vi "util.filter-rec-files-by-date.vi"(9 "Date Start":timestamp format="%<%x>T", 10 "Date End":timestamp format="%<%x>T", 11 "filenames":string[](array[string])) -> (0 "error IO":errorcluster, 3 "Array":string[](array[string]))   [LabVIEW 2024]
uses:
  <vilib>/Utility/miscctls.llb/LVDateTimeRec.ctl
panel:
  out "double precision float":dbl format="%#.0f"
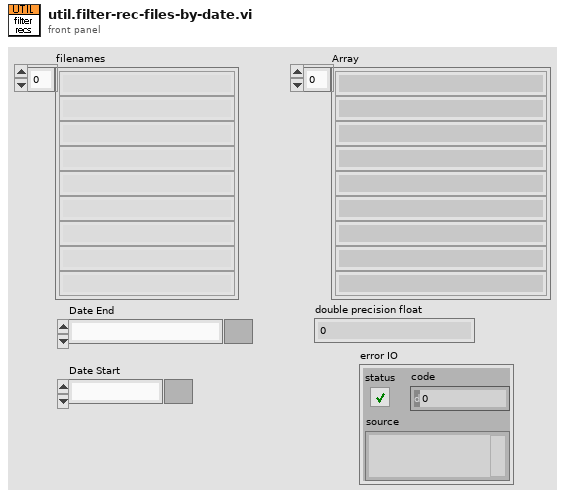
[diagram p1: front panel]
types:
  T1 = typedef "LVDateTimeRec.ctl" = cluster{"fractional second":dbl, "second":i32, "minute":i32, "hour":i32, "day of month":i32, "month":i32, "year":i32, "day of week":i32, "day of year":i32, "DST":i32}
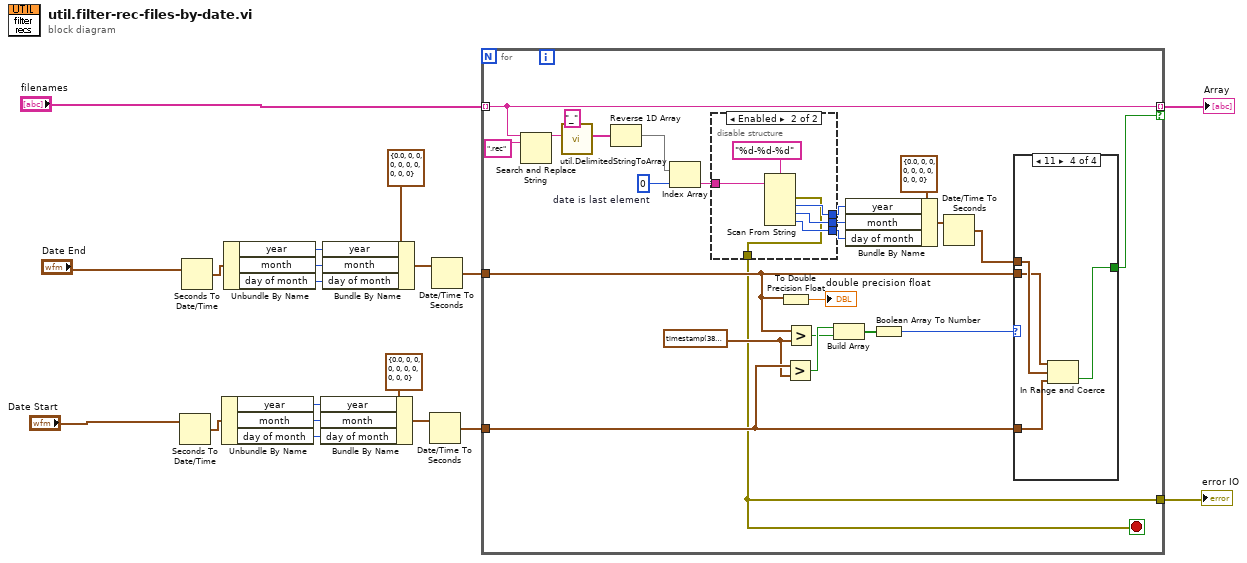
[diagram p0: block diagram]
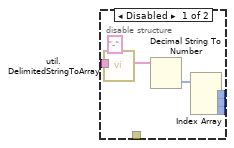
[diagram p2: hidden frame]
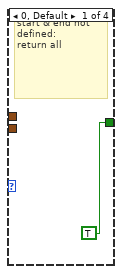
[diagram p3: hidden frame]
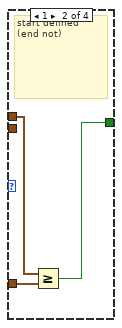
[diagram p4: hidden frame]
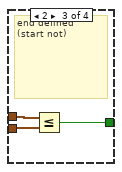
[diagram p5: hidden frame]
diagram:
  n1 = Seconds To Date/Time(time stamp (now)="Date Start") -> (date time rec=w7:T1)  [unwired: 1 in]
  n2 = Seconds To Date/Time(time stamp (now)="Date End") -> (date time rec=w14:T1)  [unwired: 1 in]
  n3 = Unbundle By Name(w7) -> ("year"=w8:i32, "month"=w9:i32, "day of month"=w10:i32)
  n4 = Unbundle By Name(w14) -> ("year"=w13:i32, "month"=w12:i32, "day of month"=w11:i32)
  n5 = Bundle By Name(cluster=T1 {"fractional second"=0.0, "second"=0, "minute"=0, "hour"=0, "day of month"=0, "month"=0, "year"=0, "day of week"=0, "day of year"=0, "DST"=0} ("date time rec"), "year"=w8, "month"=w9, "day of month"=w10) -> (w5:T1)
  n6 = Bundle By Name(cluster=T1 {"fractional second"=0.0, "second"=0, "minute"=0, "hour"=0, "day of month"=0, "month"=0, "year"=0, "day of week"=0, "day of year"=0, "DST"=0} ("date time rec"), "year"=w13, "month"=w12, "day of month"=w11) -> (w15:T1)
  n7 = Date/Time To Seconds(2:w5) -> (0:w19:timestamp)  [unwired: 1 in]
  n8 = Date/Time To Seconds(2:w15) -> (0:w18:timestamp)  [unwired: 1 in]
  n9 = for {
    tunnel: "filenames" -> [w31] mode=indexing
    tunnel: [w31] -> w3 mode=indexing if=w30
    tunnel: w18 -> [w27]
    tunnel: w19 -> [w24]
    tunnel: [w20] -> w1
    stop <- w20 stop-if-true
    w23 = timestamp(3803105846.248 s since 1904-01-01) ("Date End 2")
    w39 = 0  # date is last element
    n10 = Search and Replace String(input string=w31, search string=".rec") -> (result string=w41:string)  [unwired: 6 in, 3 out]
    n11 = call "util.DelimitedStringToArray.vi"("delimiter (,)"="_", "delimitaed string"=w41) -> ("array out"=w40:string[])  [unwired: 9 in]
    n12 = Reverse 1D Array(array=w40) -> (reversed array=w21:string[])
    n13 = Index Array(array=w21, index=w39) -> (element=w38:string)
    n14 = disable-structure shown="Enabled" {
      disable-tunnel: w38 -> [w49 w55]
      disable-tunnel: [w46 w54] -> w35
      disable-tunnel: [w45 w53] -> w34
      disable-tunnel: [w44 w52] -> w33
      disable-tunnel: [_ w51] -> w20
      frame Disabled {
        n15 = call "util.DelimitedStringToArray.vi"("delimiter (,)"="-", "delimitaed string"=w49) -> ("array out"=w48:string[])  [unwired: 9 in]
        n16 = Decimal String To Number(string=w48) -> (number=w47:i32[])  [unwired: 2 in, 1 out]
        n17 = Index Array(array=w47) -> (element #1=w46:i32, element #2=w45:i32, element #3=w44:i32)  [unwired: 3 in]
      }
      frame Enabled {
        n18 = Scan From String(format string="%d-%d-%d", input string=w55) -> (error out=w51:errorcluster, output 1=w54:i32, output 2=w53:i32, output 3=w52:i32)  [unwired: 5 in, 2 out]
      }
    }
    n19 = To Double Precision Float(number=w27) -> (double precision float=→"double precision float":dbl)
    n20 = Greater?(x=w24, y=w23) -> (0:w25:bool)
    n21 = Greater?(x=w27, y=w23) -> (0:w22:bool)
    n22 = Build Array(w25, w22) -> (w29:bool[])
    n23 = Bundle By Name(cluster=T1 {"fractional second"=0.0, "second"=0, "minute"=0, "hour"=0, "day of month"=0, "month"=0, "year"=0, "day of week"=0, "day of year"=0, "DST"=0} ("date time rec"), "year"=w35, "month"=w34, "day of month"=w33) -> (w37:T1)
    n24 = Boolean Array To Number(Boolean array=w29) -> (number=w28:u32)
    n25 = Date/Time To Seconds(2:w37) -> (0:w32:timestamp)  [unwired: 1 in]
    n26 = case shown="11" w28 {
      tunnel: w32 -> [_ w60 w63 w67]
      tunnel: w24 -> [_ w59 _ w66]
      tunnel: w27 -> [_ _ w62 w65]
      tunnel: [TRUE w58 w61 w64] -> w30
      frame 0, Default {
        # "start & end not defined:\nreturn all"
      }
      frame 1 {
        # "start defined \n(end not)"
        n27 = Greater Or Equal?(x=w60, y=w59) -> (x >= y?=w58:bool)
      }
      frame 2 {
        # "end defined\n(start not)"
        n28 = Less Or Equal?(x=w63, y=w62) -> (x <= y?=w61:bool)
      }
      frame 3 {
        n29 = In Range and Coerce(upper limit=w65, x=w67, lower limit=w66) -> (In Range?=w64:bool)  [unwired: 1 out]
      }
    }
  }
  "Array" <- w3
  "error IO" <- w1
